vi "QUDI_QPD_basic_measure.vi"() -> ()   [LabVIEW 2015]
uses:
  <vilib>/Platform/TimedLoop/XDataNode/timing_clust.ctl
  <vilib>/Platform/TimedLoop/XDataNode/nitl_modes.ctl
  <vilib>/Platform/TimedLoop/XDataNode/wakeup.ctl
  <vilib>/rvi/FXPMathLib/basic elements/FxpIntAccumulator/subVIs/nifxpmath_IntAccumulator_SimConfig.ctl
  <vilib>/rvi/Emulation/niFpgaGetClockAttributes.vi
  <vilib>/rvi/Emulation/niFpgaSctlEmulationGetInTimedLoop.vi
  <vilib>/rvi/Emulation/niFpgaEmulationReportErrorSimple.vi
  <vilib>/rvi/eio/common/nirviEmuTemplateMethod_errors.vi
  <vilib>/rvi/Emulation/niFpgaProcessEmulError.vi
  <vilib>/rvi/Analysis/common/codeGenErrors/XNode/niFpgaXNodeCodeGenErrorHandle.vi
  <vilib>/rvi/Emulation/niFpgaCriticalErrorInLSC.vi
  <vilib>/rvi/FXPMathLib/basic elements/FxpIntAccumulator/simVIs/DllFxpIntAccumulator_sub.vi
  <vilib>/eio/EIONode/EIONode.xnode
  <vilib>/rvi/Analysis/measure/dc-rms/XNode/niFpgaDC-RMS.xnode
  <vilib>/Platform/TimedLoop/XDataNode/XDataNode.xnode
  <vilib>/rvi/FXPMathLib/basic elements/FxpIntAccumulator/XNode/nifxpmath_IntAccumulator.xnode
  <vilib>/Platform/TimedLoop/XDataNode/XDNodeRunTimeDep.lvlib
panel:
  in  "ref_axis":bool
  out "counter":u32
  out "Sum":i16
  out "Y":i16
  out "X":i16
  in  "integration_time_us":u16=100 caption="Count(uSec)"
  in  "stop":bool
  out "duration_ms":u16
  in  "reset_counter":bool
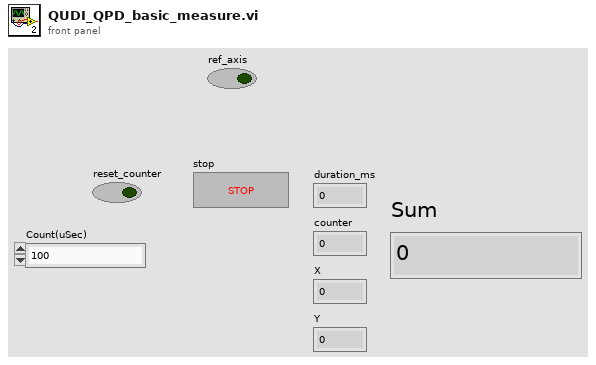
[diagram p1: front panel]
types:
  T1 = typedef "XDNodeRunTimeDep.lvlib/timing_clust.ctl" = cluster{"Expected End [f-1]":u64, "Actual End [f-1]":u64, "Finished Late? [f-1]":bool, "Expected End [i-1]":u64, "Actual End [i-1]":u64, "Finished Late? [i-1]":bool, "Expected Start [i]":u64, "Actual Start [i]":u64, "Expected Start [f]":u64, "Actual Start [f]":u64, "Source Name":string, "Structure Name":string, "Period":i64, "Deadline":i64, "Offset":i64, "Start":i64, "Priority":i32, "Timeout":i32, "Mode":T2, "Wakeup Reason":T3, "Error":errorcluster, "Source Type":string, "Secondary Source Type":string, "Global End Time":u64, "Global Start Time":u64, "Frame Duration":u64, "Iteration Duration":u64, "Assigned CPU":i32, "I/O Scan Engine Mode":u32}
  T2 = typedef "XDNodeRunTimeDep.lvlib/nitl_modes.ctl" = enum32{"No Change", "Process missed periods, maintain original phase", "Discard missed periods, maintain original phase", "Process missed periods, ignore original phase", "Discard missed periods, ignore original phase"}
  T3 = typedef "XDNodeRunTimeDep.lvlib/wakeup.ctl" = enum32{"Normal", "Aborted", "Asynchronous wakeup", "Timing source error", "Timed loop error", "Timeout"}
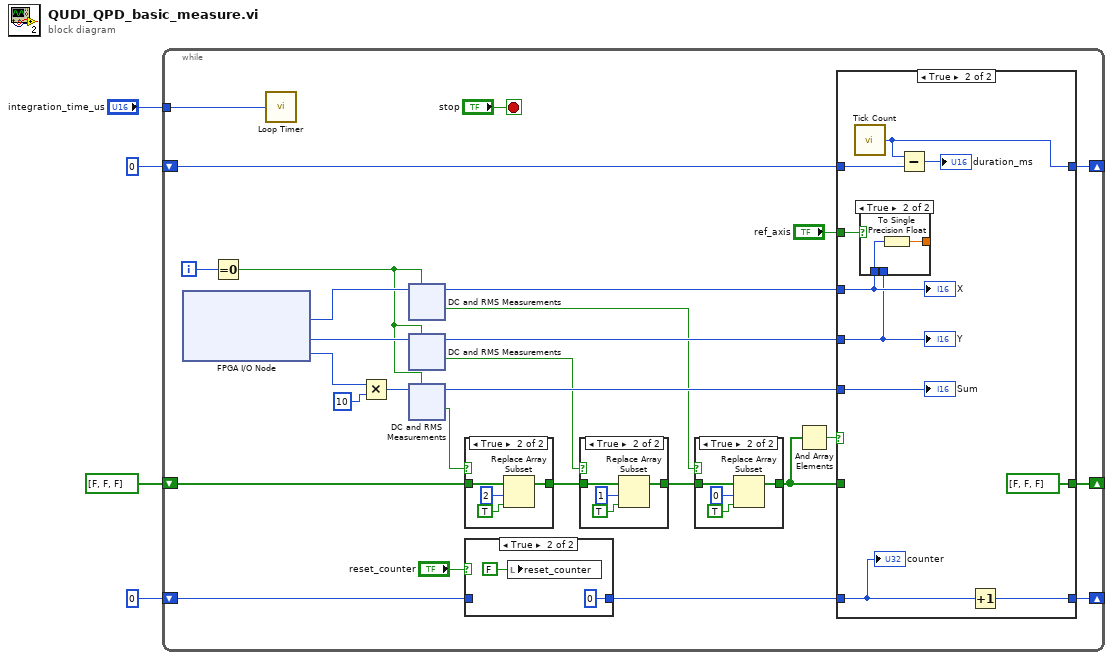
[diagram p0: block diagram]
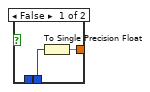
[diagram p7: hidden frame]
diagram:
  n1 = while {
    shift-right: [w16] -> _
    shift-left: bool[] [FALSE, FALSE, FALSE] ("initialized array") -> [w24]
    shift-right: [w14] -> _
    shift-left: u16 0 -> [w15]
    tunnel: "integration_time_us" -> [w13]
    shift-right: [w12] -> _
    shift-left: u32 0 -> [w10]
    i -> [w30]
    stop <- "stop" stop-if-true
    n2 = xnode "FPGA I/O Node"() -> ("Connector0/AI0"=w32:i16, "Connector0/AI1"=w28:i16, "Connector0/AI2"=w7:i16)  [unwired: 3 in, 3 out]
    n3 = Equal To 0?(x=w30) -> (x = 0?=w25:bool)
    n4 = call "Loop Timer"("Count(uSec)"=w13) -> ()  [unwired: 1 out]
    n5 = Multiply(x=w7, y=i16 10) -> (x*y=w6:i16)
    n6 = xnode "DC and RMS Measurements"("input data"=w32, "reset"=w25) -> ("DC"=w29:i16, "output valid"=w19:bool)
    n7 = xnode "DC and RMS Measurements"("input data"=w28, "reset"=w25) -> ("DC"=w27:i16, "output valid"=w20:bool)
    n8 = xnode "DC and RMS Measurements"("input data"=w6, "reset"=w25) -> ("DC"=w26:i16, "output valid"=w21:bool)
    n9 = case shown="True" w21 {
      tunnel: w24 -> [w41 w44]
      tunnel: [w41 w42] -> w23
      frame False {
      }
      frame True {
        n10 = Replace Array Subset(array=w44, new element=TRUE, index=2) -> (w42:bool[])
      }
    }
    n11 = case shown="True" "reset_counter" {
      tunnel: w10 -> [w33 _]
      tunnel: [w33 u32 0] -> w9
      frame False {
      }
      frame True {
        n12 = local write "reset_counter"(FALSE ("Reset counter")) -> ()
      }
    }
    n13 = case shown="True" w20 {
      tunnel: w23 -> [w46 w49]
      tunnel: [w46 w47] -> w22
      frame False {
      }
      frame True {
        n14 = Replace Array Subset(array=w49, new element=TRUE, index=1) -> (w47:bool[])
      }
    }
    n15 = case shown="True" w19 {
      tunnel: [w36 w38] -> w17
      tunnel: w22 -> [w36 w37]
      frame False {
      }
      frame True {
        n16 = Replace Array Subset(array=w37, new element=TRUE, index=0) -> (w38:bool[])
      }
    }
    n17 = And Array Elements(Boolean array=w17) -> (logical AND=w18:bool)
    n18 = case shown="True" w18 {
      tunnel: w29 -> [_ w55]
      tunnel: w27 -> [_ w54]
      tunnel: w26 -> [_ w58]
      tunnel: w17 -> [w53 _]
      tunnel: [w53 bool[] [FALSE, FALSE, FALSE] ("initialized array")] -> w16
      tunnel: w15 -> [w52 w62]
      tunnel: [w52 w60] -> w14
      tunnel: w9 -> [w51 w57]
      tunnel: [w51 w59] -> w12
      tunnel: "ref_axis" -> [_ w56]
      frame False {
      }
      frame True {
        n19 = call "Tick Count"() -> ("Tick Count(mSec)"=w60:u16)
        n20 = case shown="True" w56 {
          tunnel: w55 -> [_ w67]
          tunnel: [w64 w66] -> _
          tunnel: w54 -> [w65 _]
          frame False {
            n21 = To Single Precision Float(number=w65) -> (single precision float=w64:sgl)
          }
          frame True {
            n22 = To Single Precision Float(number=w67) -> (single precision float=w66:sgl)
          }
        }
        n23 = Subtract(x=w60, y=w62) -> (x-y=→"duration_ms":u16)
        n24 = Increment(x=w57) -> (x+1=w59:u32)
        "X" <- w55
        "Y" <- w54
        "Sum" <- w58
        "counter" <- w57
      }
    }
  }
